vi "tslin_switch_normal_schedule_table.vi"(8 "错误输入（无错误）":errorcluster, 9 "ASchIndex":i32, 10 "ALdxChn":i32, 11 "路径输入":path) -> (0 "错误输出":errorcluster, 2 "return":i32, 3 "路径输出":path)   [LabVIEW 2014]
doc: "Function Introduction :\nSwitch to the normal scheduling table of the specified channel\nCall location :\ninput parameter :\nAIdxChn: Channel Index\nASchIndex: Channel Index\nReturn value :\n0: Execution successful\nOther values: Failed"
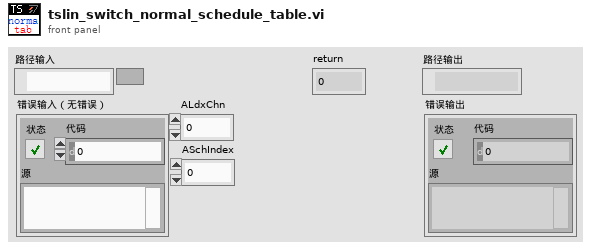
[diagram p1: front panel]
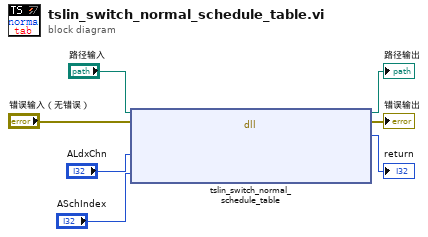
[diagram p0: block diagram]
diagram:
  n1 = dll-call lib="D:/Program Files (x86)/TOSUN/TSMaster/Data/SDK/lib/x86/TSMaster.dll" fn="tslin_switch_normal_schedule_table"(path in="路径输入", error in="错误输入（无错误）", "ALdxChn"="ALdxChn", "ASchIndex"="ASchIndex") -> (path out=→"路径输出":path, error out=→"错误输出":errorcluster, "返回类型"=→"return":i32)  [unwired: 3 in]
